vi "updateRuntime.vi"() -> ()   [LabVIEW 2012]
uses:
  <vilib>/addons/database/Auxilliary.llb/DB Tools Cursor Type.ctl
  <vilib>/addons/database/Connection.llb/DB Tools Open Connec (Path).vi
  <vilib>/addons/database/Connection.llb/Conn Execute.vi
  <vilib>/addons/database/Recordset.llb/Rec Fetch Recordset Data (R).vi
  <vilib>/addons/database/Recordset.llb/Rec Destroy - Connection.vi
  <vilib>/addons/database/Recordset.llb/Rec Fetch String Data (R).vi
  <vilib>/addons/database/_DB Variant To Data/Database Variant To Data.xnode
  <vilib>/addons/database/NI_Database_API.lvlib
panel:
  out "data 6":string
  out "data 4":string
  out "recordset data":variant[][](array[variant])
  out "concatenated string":string
  out "error out":errorcluster
  out "data 5":string
  out "data 3":i32
  out "data 2":string
  out "data":string
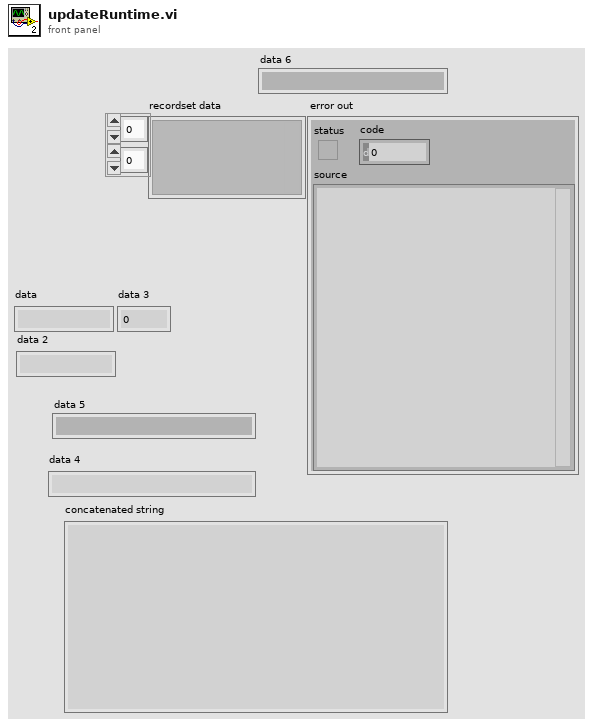
[diagram p1: front panel]
types:
  T1 = typedef "NI_Database_API.lvlib/DB Tools Cursor Type.ctl" = enum16{"forward-only", "keyset", "dynamic", "static"}
  T2 = typedef "NI_Database_API.lvlib/Conn ObjectReference.ctl" = refnum<k1>
  T3 = typedef "NI_Database_API.lvlib/Rec ObjectReference.ctl" = refnum<k1>
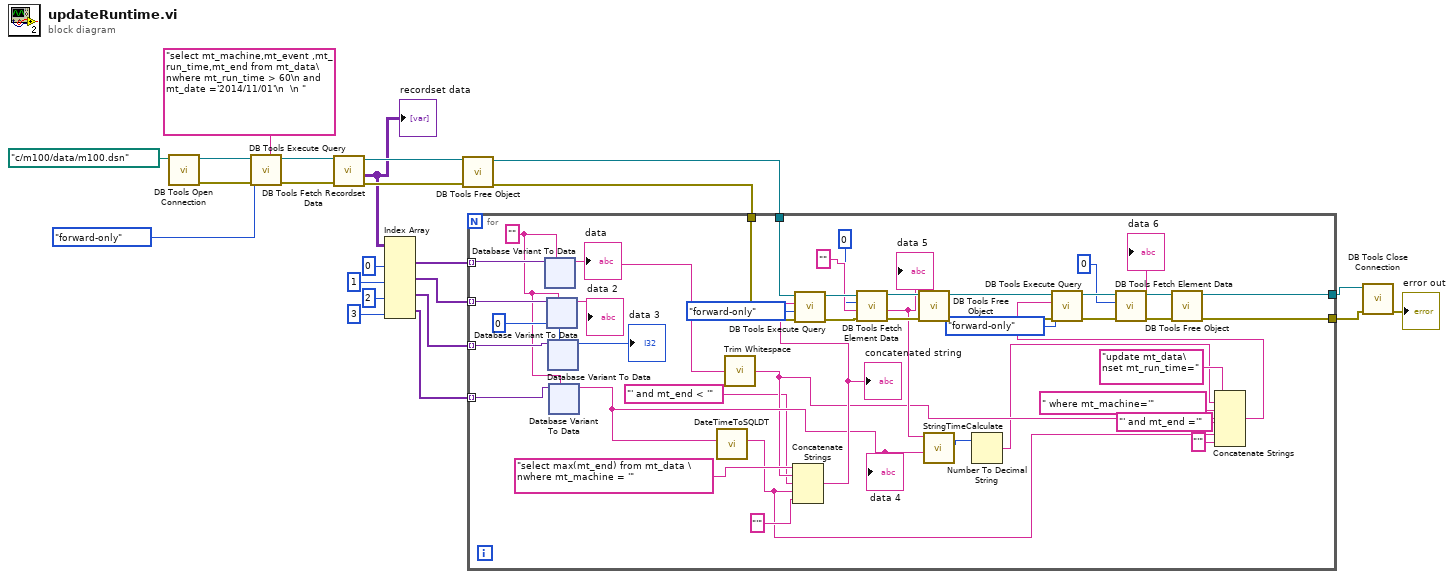
[diagram p0: block diagram]
diagram:
  n1 = call-poly <vilib>:"DB Tools Open Connection.vi"("connection information"=path "c:/m100/data/m100.dsn") -> ("error out"=w18:errorcluster, "connection reference"=w23:T2)  [unwired: 7 in]
  n2 = call-poly <vilib>:"DB Tools Execute Query.vi"("error in (no error)"=w18, "cursor type"=DB_Tools_Cursor_Type."forward-only", "SQL query"="select mt_machine,mt_event ,mt_run_time,mt_end from mt_data\nwhere mt_run_time > 60\n and mt_date ='2014/11/01'\n  \n ", "connection reference"=w23) -> ("error out"=w19:errorcluster, "recordset reference"=w22:T3)  [unwired: 4 in]
  n3 = call-poly <vilib>:"DB Tools Fetch Recordset Data.vi"("error in (no error)"=w19, "recordset reference"=w22) -> ("error out"=w20:errorcluster, "recordset data"=w3:variant[][], "recordset reference out"=w21:T3)  [unwired: 3 in]
  "recordset data" <- w3
  n4 = Index Array(array=w3, index (col) #1=0 ("disabled index (col)"), index (col) #2=1 ("index (col)"), index (col) #3=2 ("index (col)"), index (col) #4=3 ("index (col)")) -> (element #1=w10:variant[], element #2=w9:variant[], element #3=w8:variant[], element #4=w7:variant[])  [unwired: 4 in]
  n5 = call-poly <vilib>:"DB Tools Free Object.vi"("error in (no error)"=w20, "recordset reference"=w21) -> ("error out"=w5:errorcluster, "connection reference"=w6:T2)  [unwired: 8 in]
  n6 = for {
    tunnel: w10 -> [w67] mode=indexing
    tunnel: w9 -> [w66] mode=indexing
    tunnel: w8 -> [w65] mode=indexing
    tunnel: w7 -> [w64] mode=indexing
    tunnel: w6 -> [w61]
    tunnel: w5 -> [w60]
    tunnel: [w38] -> w2
    tunnel: [w37] -> w1
    w47 = ""
    n7 = xnode "Database Variant To Data"("database variant"=w67, "type"=w47) -> ("data"=w50:string)  [unwired: 1 in, 1 out]
    "data" <- w50
    n8 = xnode "Database Variant To Data"("database variant"=w66, "type"=w47) -> ("data"=→"data 2":string)  [unwired: 1 in, 1 out]
    n9 = xnode "Database Variant To Data"("database variant"=w65, "type"=0) -> ("data"=→"data 3":i32)  [unwired: 1 in, 1 out]
    n10 = xnode "Database Variant To Data"("database variant"=w64, "type"=w47) -> ("data"=w45:string)  [unwired: 1 in, 1 out]
    "data 4" <- w45
    n11 = call "DateTimeToSQLDT.vi"("DateTimeString"=w45) -> ("SQLDateTime"=w33:string)  [unwired: 10 in]
    n12 = call <vilib>:"Trim Whitespace.vi"("string"=w50) -> ("trimmed string"=w35:string)  [unwired: 1 in]
    n13 = Concatenate Strings("select max(mt_end) from mt_data \nwhere mt_machine = '" ("string"), w35, "' and mt_end < '" ("string"), w33, "'" ("string")) -> (w54:string)
    "concatenated string" <- w54
    n14 = call-poly <vilib>:"DB Tools Execute Query.vi"("error in (no error)"=w60, "cursor type"=DB_Tools_Cursor_Type."forward-only", "SQL query"=w54, "connection reference"=w61) -> ("error out"=w57:errorcluster, "recordset reference"=w59:T3)  [unwired: 4 in]
    n15 = call-poly <vilib>:"DB Tools Fetch Element Data.vi"("error in (no error)"=w57, "type"="", "column index"=0, "recordset reference"=w59) -> ("error out"=w56:errorcluster, "data"=w46:string, "recordset reference out"=w58:T3)  [unwired: 3 in]
    "data 5" <- w46
    n16 = call-poly <vilib>:"DB Tools Free Object.vi"("error in (no error)"=w56, "recordset reference"=w58) -> ("error out"=w42:errorcluster, "connection reference"=w41:T2)  [unwired: 8 in]
    n17 = call "StringTimeCalculate.vi"("End Date"=w45, "Start Date"=w46) -> ("Minutes"=w25:i32)  [unwired: 9 in]
    n18 = Number To Decimal String(number=w25) -> (decimal integer string=w24:string)  [unwired: 1 in]
    n19 = Concatenate Strings("update mt_data\nset mt_run_time=" ("string"), w24, " where mt_machine='", w35, "' and mt_end ='" ("string"), w33, "'" ("string")) -> (w31:string)
    n20 = call-poly <vilib>:"DB Tools Execute Query.vi"("error in (no error)"=w42, "cursor type"=DB_Tools_Cursor_Type."forward-only", "SQL query"=w31, "connection reference"=w41) -> ("error out"=w43:errorcluster, "recordset reference"=w40:T3)  [unwired: 4 in]
    n21 = call-poly <vilib>:"DB Tools Fetch Element Data.vi"("error in (no error)"=w43, "column index"=0, "recordset reference"=w40) -> ("error out"=w44:errorcluster, "data"=→"data 6":string, "recordset reference out"=w39:T3)  [unwired: 4 in]
    n22 = call-poly <vilib>:"DB Tools Free Object.vi"("error in (no error)"=w44, "recordset reference"=w39) -> ("error out"=w37:errorcluster, "connection reference"=w38:T2)  [unwired: 8 in]
  }
  n23 = call <vilib>:"DB Tools Close Connection.vi"("error in (no error)"=w1, "connection reference"=w2) -> ("error out"=→"error out":errorcluster)  [unwired: 5 in]
